vi "Get Default Path.vi"() -> (3 "Path":path)   [LabVIEW 2020]
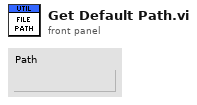
[diagram p1: front panel]
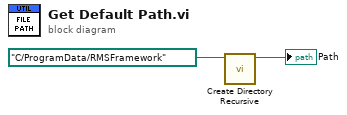
[diagram p0: block diagram]
diagram:
  n1 = call <vilib>:"Create Directory Recursive.vi"("directory"=path "C:/ProgramData/RMSFramework" ("Path")) -> ("directory copy"=→"Path":path)  [unwired: 4 in, 2 out]
